vi "DigitalIORead.vi"(3 "error in":errorcluster, 4 "Component":u16(ring) items=["left_lower_cuff", "right_lower_cuff", "left_lower_button", "right_lower_button", "left_upper_button", "right_upper_button", "left_shoulder_button", "right_shoulder_button"], 5 "node":string) -> (0 "error out":errorcluster, 1 "Digital IO State":cluster{"state":i8, "is input only":bool})   [LabVIEW 2013]
panel:
  out "Reply":string
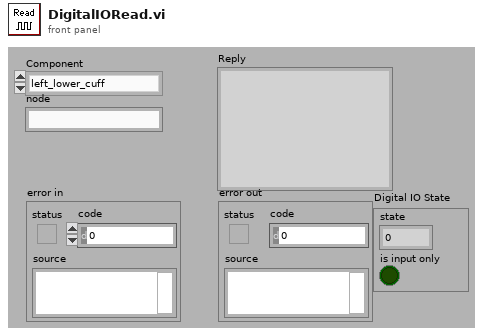
[diagram p1: front panel]
types:
  T1 = typedef "_ROSControl.ctl" = cluster{"topic port":u16, "Node":string, "topic":string, "type":string, "node port":u32, "error ":errorcluster, "Direction":T2, "APIs":string[]}
  T2 = typedef "_ROSDirection.ctl" = enum16{"Node", "Publisher", "Subscriber", "Service Client"}
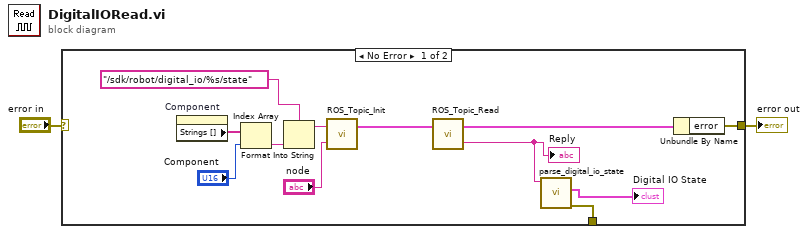
[diagram p0: block diagram]
diagram:
  n1 = case shown="No Error" "error in" {
    selector: "error in" -> [_ w15]
    tunnel: [w14 w15] -> w2
    tunnel: [w3 _] -> _
    frame No Error {
      n2 = property on="Component" class="Ring (strict)"() -> ("Strings []"=w10:string[])  [unwired: 2 in, 2 out]
      n3 = Index Array(array=w10, index="Component") -> (element=w7:string)
      n4 = Format Into String(format string="/sdk/robot/digital_io/%s/state" ("topic"), w7) -> (resulting string=w6:string)  [unwired: 2 in, 1 out]
      n5 = call "ROS_Topic_Init.vi"("node"="node", "topic"=w6) -> ("ROS out"=w12:T1)  [unwired: 1 in]
      n6 = call "ROS_Topic_Read.vi"("ROS in"=w12) -> ("Reply"=w5:string, "ROS out"=w11:T1)  [unwired: 1 in]
      "Reply" <- w5
      n7 = call "parse_digital_io_state.vi"("msg in"=w5) -> ("error out"=w3:errorcluster, "Digital IO State"=→"Digital IO State":cluster{"state":i8, "is input only":bool})  [unwired: 4 in, 1 out]
      n8 = Unbundle By Name(w11) -> ("error"=w14:errorcluster)
    }
    frame Error {
    }
  }
  "error out" <- w2
